vi "G#Object_Serialize.vi"(0 "reference in":refnum<class "G#Object.lvclass">, 1 "as xml (F)":bool, 3 "class attributes (F)":bool, 4 "object id":u32[](array[numeric]), 5 "error in (no error)":errorcluster, 7 "include aggregates (T)":bool=TRUE) -> (14 "reference out":refnum<class "G#Object.lvclass">, 16 "serialized object":string, 18 "object id out":u32[](array[numeric]), 19 "error out":errorcluster)   [LabVIEW 2020, in "G#Object.lvclass"]
doc: "Serializes the object to a binary or xml string.\n\nNotice: Serialization of aggregates using XML is not supported!"
uses:
  G#Object.lvclass
  utils/G#Object_State.ctl
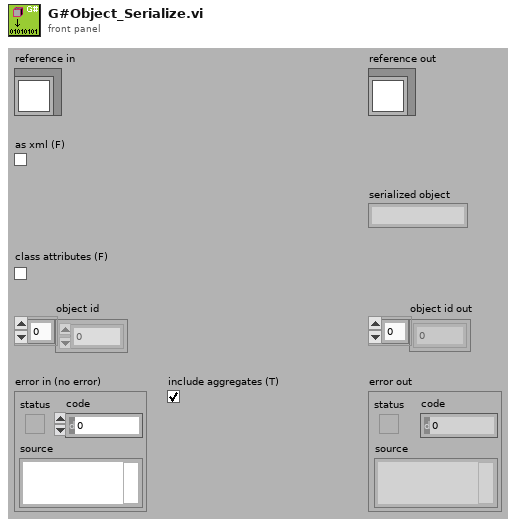
[diagram p1: front panel]
types:
  T1 = typedef "G#Object.lvclass/G#Object_State.ctl" = enum16{"Clear", "Create", "Delete", "Get class attributes", "Class hierarchy", "Get attribute value", "Set attribute value"}
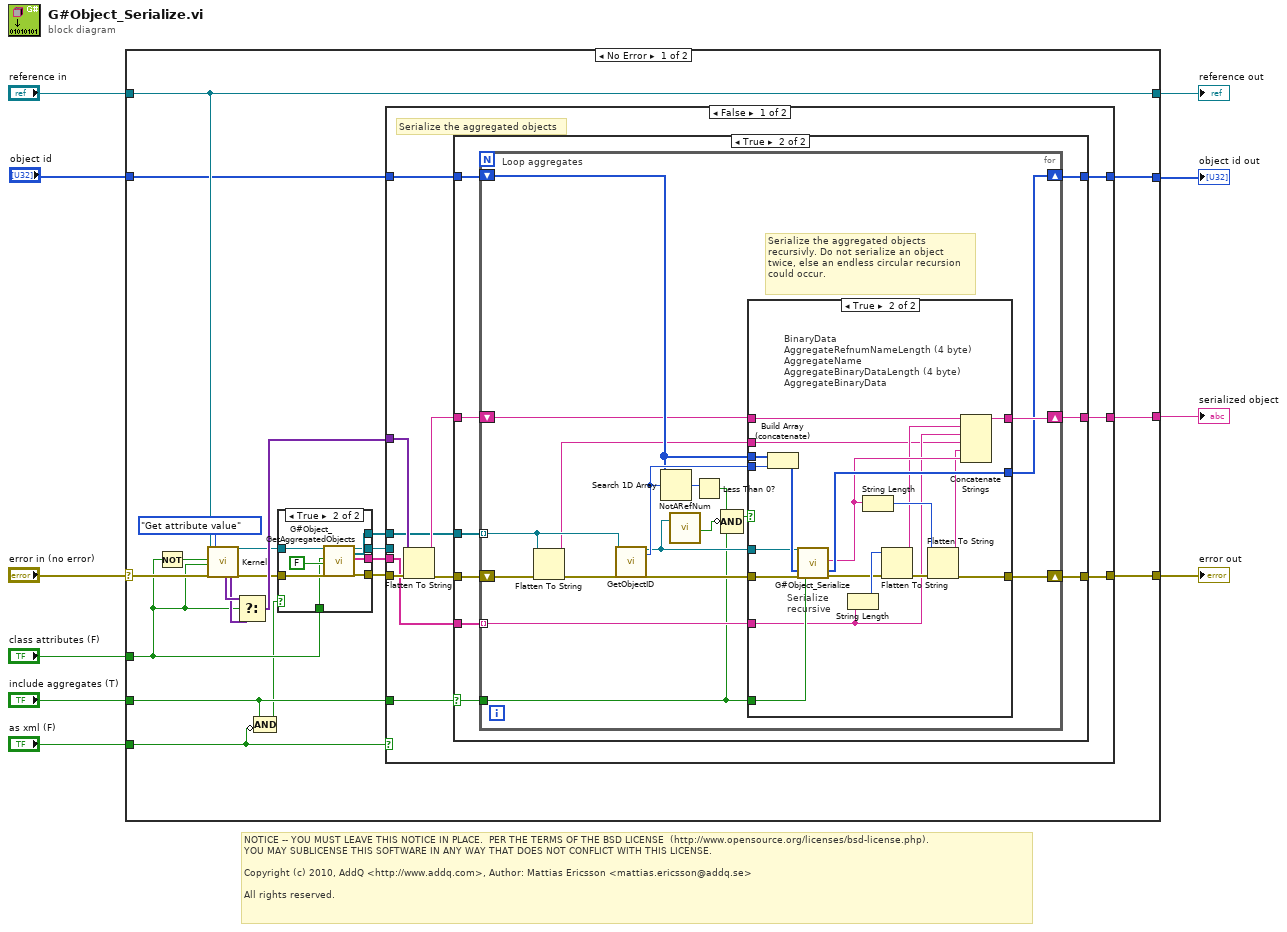
[diagram p0: block diagram]
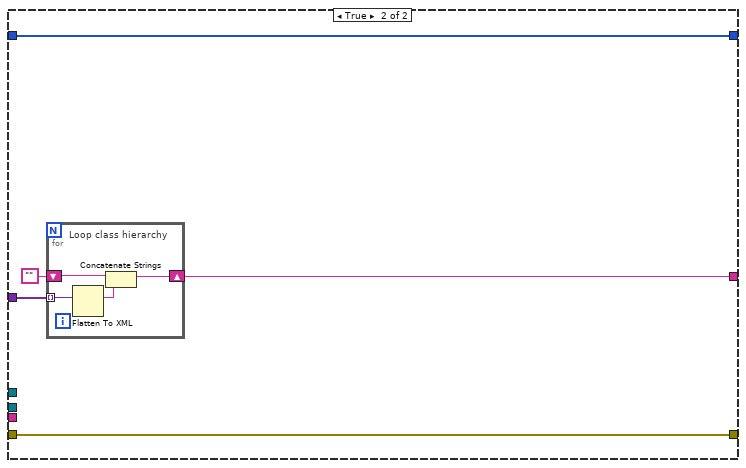
[diagram p5: hidden frame]
diagram:
  # "NOTICE -- YOU MUST LEAVE THIS NOTICE IN PLACE.  PER THE TERMS OF THE BSD LICENSE  (http://www.opensource.org/licenses/bsd-license.php).\nYOU MAY SUBLICENSE THIS SOFTWARE IN ANY WAY THAT DOES NOT CONFLICT WITH THIS LICENSE.\n\nCopyright (c) 2010, AddQ <http://www.addq.com>, Author: Mattias Ericsson <mattias.ericsson@addq.se>\n\nAll rights reserved."
  n1 = case shown="No Error" "error in (no error)" {
    selector: "error in (no error)" -> [w31 w116]
    tunnel: [w17 w116] -> w9
    tunnel: [w25 w115] -> w7
    tunnel: "reference in" -> [w25 w115]
    tunnel: [w18 _] -> w6
    tunnel: "class attributes (F)" -> [w14 _]
    tunnel: "as xml (F)" -> [w13 _]
    tunnel: "object id" -> [w19 w114]
    tunnel: [w16 w114] -> w2
    tunnel: "include aggregates (T)" -> [w12 _]
    frame No Error {
      n2 = Not(x=w14) -> (.not. x?=w26:bool)
      n3 = call-dynamic "Kernel.vi"("reference in"=w25, "option 1"=w26, "option 2"=w14, "error in (no error)"=w31, "state"=G#Object_State."Get attribute value" ("State")) -> ("class attributes out"=w29:variant[], "attributes out"=w28:variant[], "reference out"=w23:refnum<class "G#Object.lvclass">, "error out"=w24:errorcluster)  [unwired: 6 in, 5 out]
      n4 = Select(t=w29, s=w14, f=w28) -> (s? t:f=w27:variant[])
      n5 = Compound Arithmetic op=AND(w12, invert w13) -> (w11:bool)
      n6 = case shown="True" w11 {
        tunnel: w24 -> [w32 w41]
        tunnel: w23 -> [w33 w40]
        tunnel: [w32 w39] -> w22
        tunnel: [_ w38] -> w21
        tunnel: [_ w37] -> w20
        tunnel: [w33 w35] -> w15
        tunnel: w14 -> [_ w34]
        frame False {
        }
        frame True {
          n7 = call "G#Object_GetAggregatedObjects.vi"("reference in"=w40, "class attributes (F)"=w34, "array names (T)"=FALSE, "error in (no error)"=w41) -> ("reference out"=w35:refnum<class "G#Object.lvclass">, "aggregated objects"=w38:refnum<class "G#Object.lvclass">[], "aggregated names"=w37:string[], "error out"=w39:errorcluster)  [unwired: 12 in]
        }
      }
      n8 = case shown="False" w13 {
        tunnel: w22 -> [w52 w105]
        tunnel: [w47 w105] -> w17
        tunnel: [w48 w107] -> w18
        tunnel: w27 -> [w51 w109]
        tunnel: w21 -> [w46 _]
        tunnel: w20 -> [w42 _]
        tunnel: w12 -> [w45 _]
        tunnel: w19 -> [w44 w106]
        tunnel: [w43 w106] -> w16
        tunnel: w15 -> [_ _]
        frame False {
          # "Serialize the aggregated objects"
          n9 = Flatten To String(anything=w51, error in (no error)=w52) -> (data string=w50:string, error out=w49:errorcluster)  [unwired: 2 in, 1 out]
          n10 = case shown="True" w45 {
            selector: w45 -> [_ w57]
            tunnel: w50 -> [w55 w64]
            tunnel: w49 -> [w54 w63]
            tunnel: [w55 w62] -> w48
            tunnel: [w54 w61] -> w47
            tunnel: w46 -> [_ w60]
            tunnel: w44 -> [w53 w59]
            tunnel: [w53 w58] -> w43
            tunnel: w42 -> [_ w56]
            frame False {
            }
            frame True {
              n11 = for {
                shift-right: [w74] -> w61
                shift-left: w63 -> [w82]
                shift-right: [w75] -> w62
                shift-left: w64 -> [w70]
                tunnel: w60 -> [w71] mode=indexing
                shift-right: [w72] -> w58
                shift-left: w59 -> [w73]
                tunnel: w57 -> [w66]
                tunnel: w56 -> [w69] mode=indexing
                # "Loop aggregates"
                # "Serialize the aggregated objects\nrecursivly. Do not serialize an object\ntwice, else an endless circular recursion\ncould occur."
                n12 = Flatten To String(anything=w71, error in (no error)=w82) -> (data string=w68:string, error out=w81:errorcluster)  [unwired: 2 in, 1 out]
                n13 = call-dynamic "GetObjectID.vi"("reference in"=w71, "error in (no error)"=w81) -> ("reference out"=w67:refnum<class "G#Object.lvclass">, "object ID"=w80:u32, "error out"=w79:errorcluster)  [unwired: 15 in]
                n14 = Search 1D Array(1D array=w73, element=w80) -> (index of element=w78:i32)  [unwired: 1 in]
                n15 = call-dynamic "NotARefNum.vi"("reference in"=w67) -> ("not a refnum?"=w65:bool)  [unwired: 1 in, 1 out]
                n16 = Less Than 0?(x=w78) -> (x < 0?=w77:bool)
                n17 = Compound Arithmetic op=AND(w77, invert w65, w66) -> (w76:bool)
                n18 = case shown="True" w76 {
                  tunnel: w70 -> [w85 w104]
                  tunnel: [w83 w95] -> w74
                  tunnel: [w85 w103] -> w75
                  tunnel: w80 -> [_ w101]
                  tunnel: w73 -> [w84 w102]
                  tunnel: w67 -> [_ w99]
                  tunnel: w79 -> [w83 w98]
                  tunnel: [w84 w97] -> w72
                  tunnel: w66 -> [_ w96]
                  tunnel: w69 -> [_ w88]
                  tunnel: w68 -> [_ w86]
                  frame False {
                    # "Do not serialize\na dead or already\nserialized object"
                  }
                  frame True {
                    # "BinaryData\nAggregateRefnumNameLength (4 byte)\nAggregateName\nAggregateBinaryDataLength (4 byte)\nAggregateBinaryData"
                    # "Serialize\nrecursive"
                    n19 = Build Array (concatenate)(w102, w101) -> (w100:u32[])
                    n20 = call-dynamic "G#Object_Serialize.vi"("reference in"=w99, "object id"=w100, "error in (no error)"=w98, "include aggregates (T)"=w96) -> ("serialized object"=w93:string, "object id out"=w97:u32[], "error out"=w90:errorcluster)  [unwired: 12 in, 1 out]
                    n21 = String Length(string=w88) -> (length=w91:i32)
                    n22 = String Length(string=w93) -> (length=w94:i32)
                    n23 = Flatten To String(anything=w91, error in (no error)=w90) -> (data string=w89:string, error out=w92:errorcluster)  [unwired: 2 in, 1 out]
                    n24 = Flatten To String(anything=w94, error in (no error)=w92) -> (data string=w87:string, error out=w95:errorcluster)  [unwired: 2 in, 1 out]
                    n25 = Concatenate Strings(w104, w89, w88, w86, w87, w93) -> (w103:string)
                  }
                }
              }
            }
          }
        }
        frame True {
          n26 = for {
            tunnel: w109 -> [w113] mode=indexing
            shift-right: [w111] -> w107
            shift-left: "" -> [w112]
            # "Loop class hierarchy"
            n27 = Flatten To XML(6:w113) -> (2:w110:string)
            n28 = Concatenate Strings(w112, w110) -> (w111:string)
          }
        }
      }
    }
    frame Error {
    }
  }
  "error out" <- w9
  "reference out" <- w7
  "serialized object" <- w6
  "object id out" <- w2
